vi "L0_Sum_Adder.vi"() -> ()   [LabVIEW 2009]
uses:
  <instrlib>/Agilent 8000 Series/Public/Configure/Configure Math (Binary Operation).vi
  <vilib>/Utility/file.llb/Write To Spreadsheet File (string).vi
  <instrlib>/Agilent 8000 Series/Public/Data/Low Level/Fetch Measurement (More).vi
  <instrlib>/Agilent 8000 Series/Agilent 8000 Series.lvlib
panel:
  out "error out":errorcluster
  in  "Voltage Array":dbl[](array[numeric])=[0.2, 0.4, 0.6, 0.8]
  in  "Channels Combinations":i32[](array[numeric])=[3, 12, 48, 96, 7, 28, 112, 15, 120, 31, 124, 63, 126, 127]
  in  "NChannels":i32[](array[numeric])=[2, 2, 2, 2, 3, 3, 3, 4, 4, 5, 5, 6, 6, 7]
  in  "Osc":refnum<visa-resource-name>="Oscilloscope"
  in  "Generator":refnum<visa-resource-name>="Generator_1"
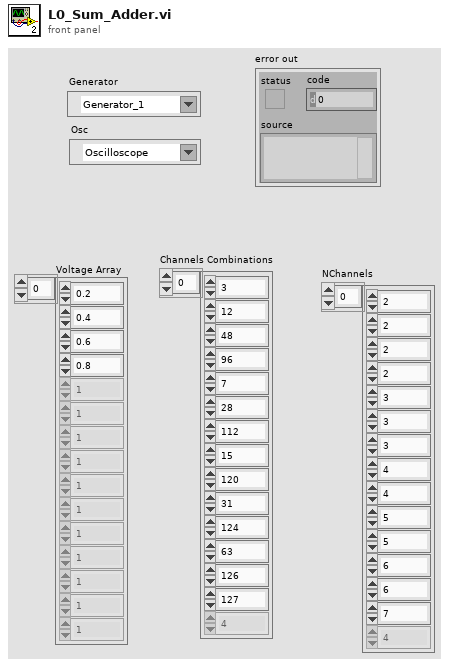
[diagram p1: front panel]
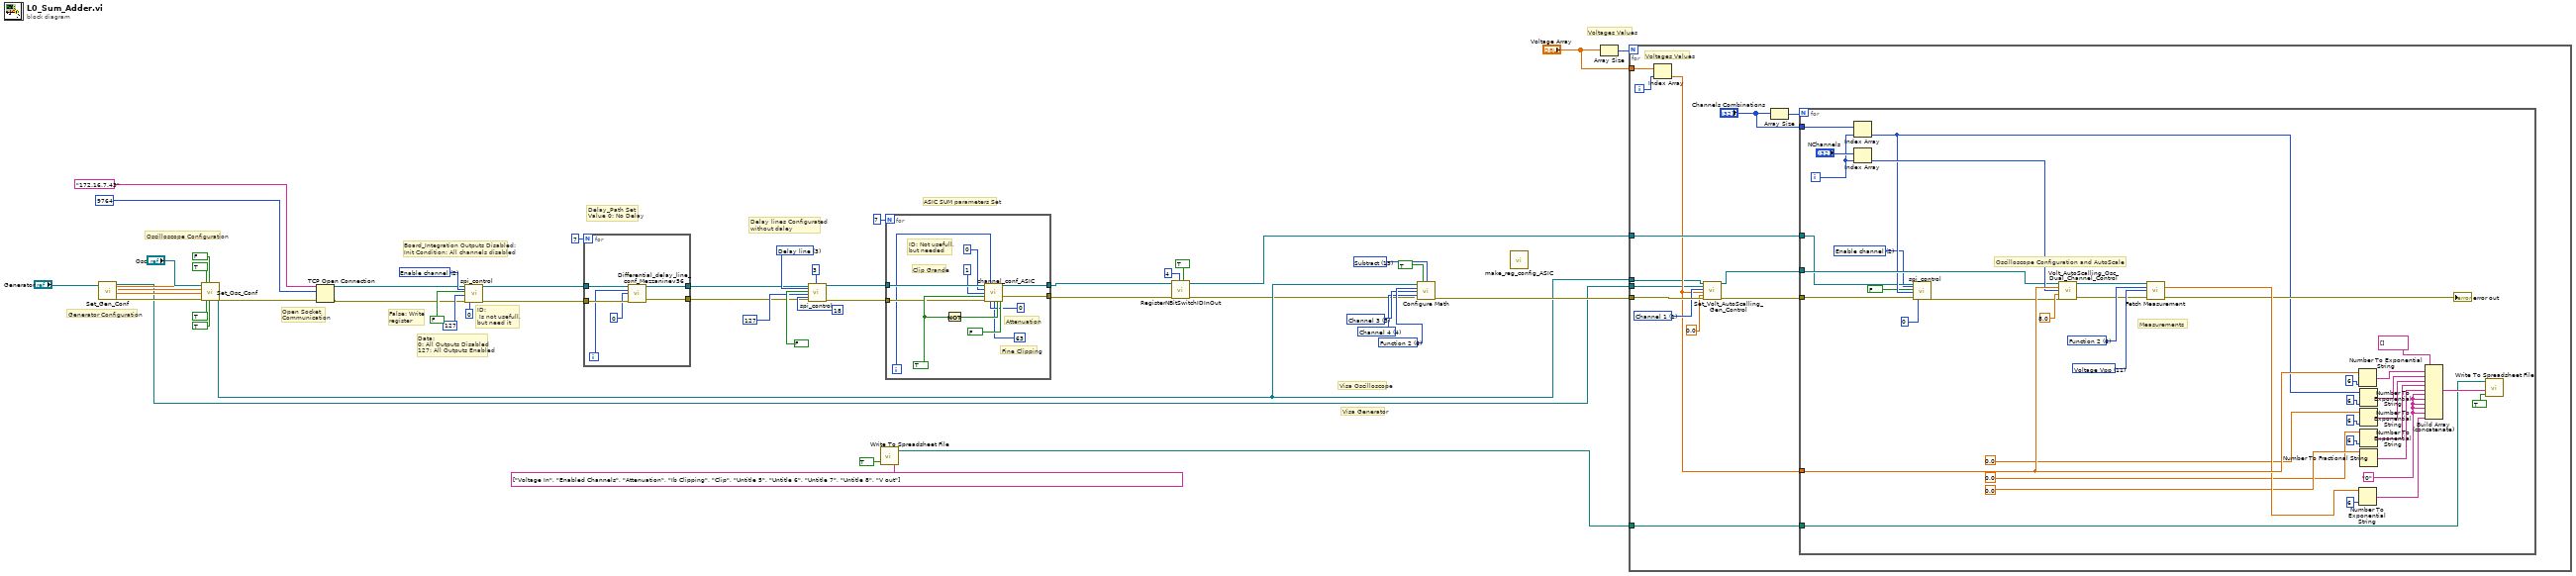
[diagram p0: block diagram]
diagram:
  w20 = u16 2 items=["Attenuation", "Clipping", "Enable channel", "Delay line", "ASIC"] ("Device")
  w23 = u16 3 items=["Attenuation", "Clipping", "Enable channel", "Delay line", "ASIC"] ("Device")
  w35 = u16 6 items=["Function 1"=5, "Function 2"=6, "Function 3"=7, "Function 4"=8] ("Math Channel (5: Function 1)")
  w36 = u16 15 items=["Add"=12, "Divide"=13, "Multiply"=14, "Subtract"=15, "Common Mode"=16, "Versus"=17] ("Math Operation (12: Add)")
  w34 = 3 items=["Channel 1"=1, "Channel 2"=2, "Channel 3"=3, "Channel 4"=4] ("Channel (1: Channel 1)")
  w33 = 4 items=["Channel 1"=1, "Channel 2"=2, "Channel 3"=3, "Channel 4"=4] ("Channel (1: Channel 1)")
  # "ASIC SUM parameters Set"
  # "Delay_Path Set\nValue 0: No Delay"
  # "False: Write\nregister"
  # "Data:\n0: All Outputs Disabled\n127: All Outputs Enabled"
  # "ID:\n Is not usefull, \nbut need it"
  # "Board_Integration Outputs Disabled:\nInit Condition: All channels disabled"
  # "Delay lines Configurated \nwithout daley"
  # "Open Socket\nCommunication"
  # "Visa Generator"
  # "Visa Oscilloscope"
  # "Oscilloscope Configuration"
  # "Voltages Values"
  # "Generator Configuration"
  n1 = call "Set_Gen_Conf.vi"("AWG VISA"="Generator") -> ("Amplitude 1 OUT"=w43:dbl, "VISA resource name out"=w28:refnum<visa-resource-name>, "Pulse Width in seconds 1 OUT"=w42:dbl, "Trigger Level 1"=w41:dbl, "error out"=w40:errorcluster)  [unwired: 11 in, 3 out]
  n2 = call "Set_Osc_Conf.vi"("VISA resource name"="Osc", "Amplitude IN"=w43, "Trigger Level IN"=w41, "Pulse Width in seconds IN"=w42, "error in (no error)"=w40, "Channel 1"=TRUE, "Channel 3"=TRUE, "Channel 2"=FALSE, "Channel 4"=TRUE) -> ("VISA resource name out"=w27:refnum<visa-resource-name>, "error out"=w17:errorcluster)  [unwired: 9 in]
  n3 = TCP Open Connection(address="172.16.7.43", remote port or service name=u16 9764, error in (no error)=w17) -> (connection ID=w11:refnum<k5>, error out=w10:errorcluster)  [unwired: 2 in]
  n4 = call "spi_control.vi"("connection ID"=w11, "Device"=w20, "Read/#write"=FALSE, "Data"=127, "error out 3"=w10, "Id in"=0) -> ("connection ID out"=w16:refnum<k5>, "error out 2"=w15:errorcluster)  [unwired: 6 in, 6 out]
  n5 = for {
    N: 7 -> [_]
    tunnel: w15 -> [w57]
    tunnel: w16 -> [w56]
    tunnel: [w55] -> w14
    tunnel: [w54] -> w13
    i -> [w53]
    n6 = call "Differential_delay_line_conf_Mezzaninev56.vi"("connection ID"=w56, "channel"=w53, "Delay value"=u16 0, "error in (no error)"=w57) -> ("connection ID out"=w55:refnum<k5>, "error out 2"=w54:errorcluster)  [unwired: 4 in, 6 out]
  }
  n7 = call "spi_control.vi"("connection ID"=w14, "Device"=w23, "Read/#write"=FALSE, "Data"=127, "Register or channel"=18, "error out 3"=w13, "chip delay"=3) -> ("connection ID out"=w8:refnum<k5>, "error out 2"=w9:errorcluster)  [unwired: 5 in, 6 out]
  n8 = call-poly <vilib>:"Write To Spreadsheet File.vi"("append to file? (new file:F)"=TRUE, "1D data"=string[] ["Voltage In", "Enabled Channels", "Attenuation", "Ib Clipping", "Clip", "Untitle 5", "Untitle 6", "Untitle 7", "Untitle 8", "V out"]) -> ("new file path (Not A Path if cancelled)"=w29:path)  [unwired: 6 in]
  n9 = for {
    N: 7 -> [_]
    tunnel: w9 -> [w66]
    tunnel: w8 -> [w65]
    tunnel: [w64] -> w4
    tunnel: [w59] -> w7
    i -> [w62]
    w68 = TRUE ("maj/sum")
    # "Attenuation"
    # "Fine Clipping"
    # "Clip Grande"
    # "ID: Not usefull,\nbut needed"
    n10 = Not(x=w68) -> (.not. x?=w67:bool)
    n11 = call "channel_conf_ASIC.vi"("connection ID"=w65, "Ring"=w62, "Id in"=u32 0, "Clip_sel_b"=u32 1, "CompBuf_en_b"=w68, "error out"=w66, "Att gain"=u32 0, "Ib_ClipVb"=u32 63, "Clip_en_b"=w67, "Att_en_b"=FALSE) -> ("connection ID out"=w64:refnum<k5>, "error out 2"=w59:errorcluster)  [unwired: 1 in, 3 out]
  }
  n12 = call "RegisterNBitSwitchIDInOut.vi"("Switch Bit"=TRUE, "N Bit"=u16 4, "error in (no error)"=w7, "connection ID"=w4) -> ("error out"=w5:errorcluster, "connection ID out"=w3:refnum<k5>)  [unwired: 5 in]
  n13 = call-poly <instrlib>:"Configure Math.vi"("VISA resource name"=w27, "Enable Math Channel (T:Enable)"=TRUE, "Math Operation (12: Add)"=w36, "Math Channel (5: Function 1)"=w35, "Math Operand (1: Channel 1)"=w34, "Math Operand (2: Channel 2)"=w33, "error in (no error)"=w5) -> ("error out"=w32:errorcluster)  [unwired: 7 in, 1 out]
  n14 = call "make_reg_config_ASIC.vi"() -> ()  [unwired: 6 in, 1 out]
  n15 = Array Size(array="Voltage Array") -> (size(s)=w39:i32)
  n16 = for {
    N: w39 -> [_]
    tunnel: w3 -> [w76]
    tunnel: w32 -> [w79]
    tunnel: "Voltage Array" -> [w83]
    tunnel: w29 -> [w74]
    tunnel: w28 -> [w72]
    tunnel: w27 -> [w71]
    i -> [w82]
    w78 = 1 items=["Channel 1"=1, "Channel 2"=2, "Channel 3"=3, "Channel 4"=4] ("Channel")
    # "Voltages Values"
    n17 = Index Array(array=w83, index=w82) -> (element=w75:dbl)
    n18 = call "Set_Volt_AutoScalling_Gen_Control.vi"("VISA Oscilloscope"=w71, "VISA Generator"=w72, "Channel"=w78, "Amplitude"=w75, "DC Offset"=0.0, "error in (no error)"=w79) -> ("VISA Oscilloscope"=w70:refnum<visa-resource-name>, "error out"=w77:errorcluster)  [unwired: 11 in, 1 out]
    n19 = Array Size(array="Channels Combinations") -> (size(s)=w81:i32)
    n20 = for {
      N: w81 -> [_]
      tunnel: "Channels Combinations" -> [w122]
      tunnel: w77 -> [w93]
      tunnel: w76 -> [w91]
      tunnel: w75 -> [w101]
      tunnel: w74 -> [w102]
      tunnel: w70 -> [w98]
      i -> [w120]
      w89 = u16 2 items=["Attenuation", "Clipping", "Enable channel", "Delay line", "ASIC"] ("Device")
      w108 = "0" ("F-format string")
      w118 = 11 items=["Rise Time", "Fall Time", "Frequency", "Period", "Voltage RMS(AC)", "Voltage RMS(DC)", "Voltage RMS (AC,cycle)", "Voltage RMS (DC,cycle)", "Voltage Max", "Voltage Min", "Voltage Middle", "Voltage Vpp", "Voltage High", "Voltage Low", "Voltage Average", "Voltage Average (cycle)", "Width Negative", "Width Positive", "Duty Cycle Positive", "Amplitude", "Overshoot", "Preshoot", "Voltage Base", "Voltage Upper", "Time Max", "Time Min", "Color Grade Crossing", "Color Grade Eye Width", "Color Grade Eye Height", "Color Grade Eye Q-Factory", "Color Grade Eye Duty Cycle Distortion(Percent)", "Color Grade Eye Duty Cycle Distortion(Time)", "Color Grade Eye Jitter(PP)", "Color Grade Eye Width(RMS)", "Cycle-cycle Duty Jitter(Rising)", "Cycle-cycle Duty Jitter(Falling)", "Cycle-cycle Jitter(Rising)", "Cycle-cycle Jitter(Falling)", "Cycle-cycle - Width", "Cycle-cycle + Width", "Date Rate", "Unit Interval", "FFT Delta Frequency", "FFT Delta Magnitude", "FFT Frequency", "FFT Magnitude", "Slew Rate", "Area (Entire Display)", "Area(Single Cycle)", "Duty Cycle (Rising)", "Duty Cycle (Falling)"] ("Measurement Function (0: Rise Time)")
      w119 = 6 items=["Channel 1"=1, "Channel 2"=2, "Channel 3"=3, "Channel 4"=4, "Function 1"=5, "Function 2"=6, "Function 3"=7, "Function 4"=8, "Memory 1"=9, "Memory 2"=10, "Memory 3"=11, "Memory 4"=12] ("Channel (1: Channel 1)")
      # "Measurements"
      # "Oscilloscope Configuration and AutoScale"
      n21 = Index Array(array=w122, index=w120) -> (element=w92:i32)
      n22 = Index Array(array="NChannels", index=w120) -> (element=w100:i32)
      n23 = call "spi_control.vi"("connection ID"=w91, "Device"=w89, "Read/#write"=FALSE, "Data"=w92, "error out 3"=w93, "Id in"=0) -> ("error out 2"=w88:errorcluster)  [unwired: 6 in, 7 out]
      n24 = call "Volt_AutoScalling_Osc_Dual_Channel_Control.vi"("VISA Oscilloscope"=w98, "Voltage In"=w101, "N Channels"=w100, "Offset Divider"=8.0, "error in"=w88) -> ("VISA resource name out"=w97:refnum<visa-resource-name>, "error out"=w95:errorcluster)  [unwired: 9 in]
      n25 = call-poly <instrlib>:"Fetch Measurement.vi"("VISA resource name"=w97, "Channel (1: Channel 1)"=w119, "Measurement Function (0: Rise Time)"=w118, "error in (no error)"=w95) -> ("Measurement"=w96:dbl, "error out"=→"error out":errorcluster)  [unwired: 9 in, 1 out]
      n26 = Number To Exponential String(number=w101, precision (6)=i16 6) -> (E-format string=w109:string)  [unwired: 2 in]
      n27 = Number To Exponential String(number=w96, precision (6)=i16 6) -> (E-format string=w107:string)  [unwired: 2 in]
      n28 = Number To Exponential String(number=w92, precision (6)=i16 6) -> (E-format string=w117:string)  [unwired: 2 in]
      n29 = Number To Exponential String(number=0.0 ("Offset Divider"), precision (6)=i16 6) -> (E-format string=w116:string)  [unwired: 2 in]
      n30 = Number To Exponential String(number=0.0 ("Offset Divider"), precision (6)=i16 6) -> (E-format string=w114:string)  [unwired: 2 in]
      n31 = Number To Fractional String(number=0.0 ("Offset Divider")) -> (F-format string=w110:string)  [unwired: 3 in]
      n32 = Build Array (concatenate)(string[] [] ("array"), w109, w117, w116, w114, w110, w108, w108, w108, w108, w108, w107) -> (w103:string[])
      n33 = call-poly <vilib>:"Write To Spreadsheet File.vi"("append to file? (new file:F)"=TRUE, "1D data"=w103, "file path (dialog if empty)"=w102) -> ()  [unwired: 5 in, 1 out]
    }
  }
